vi "PQresStatus.vi"(8 "error in (no error)":errorcluster, 11 "status":i64) -> (0 "error out":errorcluster, 3 "return type":string)   [LabVIEW 2019, in "libpqlv64.lvlib"]
doc: "Converts the enumerated type returned by PQresultStatus into a string constant describing the status code. The caller should not free the result."
uses:
  libpqlv64.lvlib
  libpq.dll
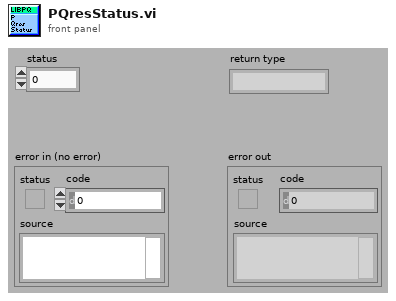
[diagram p1: front panel]
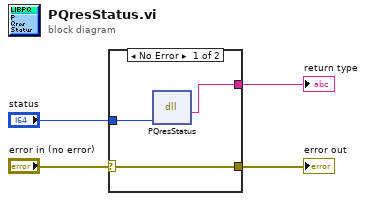
[diagram p0: block diagram]
diagram:
  n1 = case shown="No Error" "error in (no error)" {
    selector: "error in (no error)" -> [w7 w8]
    tunnel: [w7 w8] -> w3
    tunnel: [w6 _] -> w2
    tunnel: "status" -> [w5 _]
    frame No Error {
      n2 = dll-call lib="libpq.*" fn="PQresStatus"("status"=w5) -> ("return type"=w6:string)  [unwired: 4 in, 2 out]
    }
    frame Error {
    }
  }
  "return type" <- w2
  "error out" <- w3
